vi "Create Pattern Script.vi"(5 "NumofCycleRd":u32, 6 "Period(ms)":dbl format="%#_13g", 7 "Wait(ms)":dbl format="%#_13g", 8 "error in (no error)":errorcluster, 9 "Protocol Type":T1, 10 "Config Array":string[](array[string]), 11 "Protocol Interface in":refnum<class "Protocol Interface.lvclass">) -> (0 "error out":errorcluster, 2 "Pattern Script out":string, 3 "Protocol Interface out":refnum<class "Protocol Interface.lvclass">)   [LabVIEW 2018, in "Protocol Interface.lvlib" / "Protocol Interface.lvclass"]
uses:
  Protocol Interface.lvclass
  Ctls/Protocol Type.ctl
  Protocol Interface.lvclass/Protocol Interface.ctl
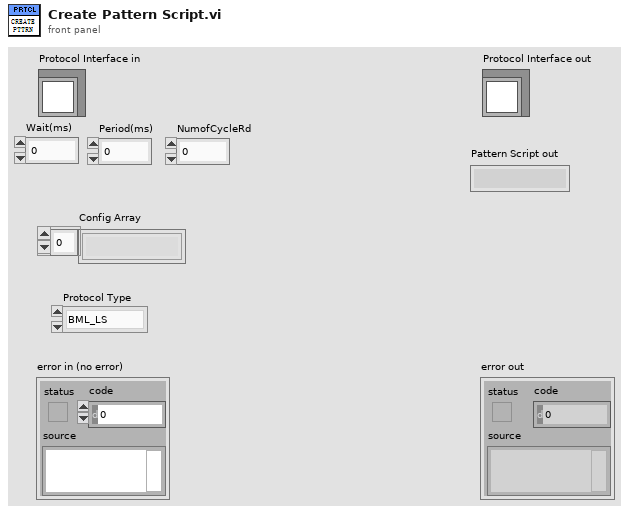
[diagram p1: front panel]
types:
  T1 = typedef "Protocol Type.ctl" = enum16{"BML_LS", "BML_HS", "SPI_3W", "SPI_4W"}
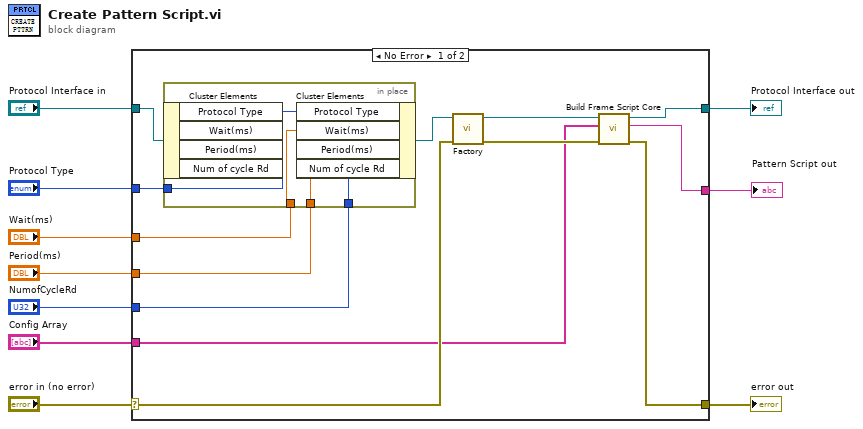
[diagram p0: block diagram]
diagram:
  n1 = case shown="No Error" "error in (no error)" {
    selector: "error in (no error)" -> [w20 w29]
    tunnel: [w17 w29] -> w9
    tunnel: [w19 w28] -> w7
    tunnel: "Protocol Interface in" -> [w23 w28]
    tunnel: "Protocol Type" -> [w22 _]
    tunnel: "Config Array" -> [w12 _]
    tunnel: [w18 _] -> w4
    tunnel: "Wait(ms)" -> [w14 _]
    tunnel: "Period(ms)" -> [w13 _]
    tunnel: "NumofCycleRd" -> [w11 _]
    frame No Error {
      n2 = in-place {
        in-place-border: w22 -> [w27]
        in-place-border: w14 -> [w26]
        in-place-border: w13 -> [w25]
        in-place-border: w11 -> [w24]
        n3 = in-place-cluster #1(w23) -> ()  [unwired: 4 out]
        n4 = in-place-cluster #1("Protocol Type"=w27, "Wait(ms)"=w26, "Period(ms)"=w25, "Num of cycle Rd"=w24) -> (w21:refnum<class "Protocol Interface.lvclass">)
      }
      n5 = call "Factory.vi"("error in (no error)"=w20, "Protocol Interface in"=w21) -> ("error out"=w15:errorcluster, "Protocol Interface out"=w16:refnum<class "Protocol Interface.lvclass">)  [unwired: 8 in]
      n6 = call-dynamic "Build Frame Script Core.vi"("error in (no error)"=w15, "Config Array"=w12, "Protocol Interface in"=w16) -> ("error out"=w17:errorcluster, "Pattern Script"=w18:string, "Protocol Interface out"=w19:refnum<class "Protocol Interface.lvclass">)  [unwired: 6 in]
    }
    frame Error {
    }
  }
  "error out" <- w9
  "Protocol Interface out" <- w7
  "Pattern Script out" <- w4
